vi "Helm Adjust Headings for PID.vi"(8 "error in (no error)":errorcluster, 11 "RDS Helm Actor in":refnum<class "RDS Helm Actor.lvclass">) -> (0 "error out":errorcluster, 1 "Current Position":dbl, 2 "Setpoint":dbl, 3 "RDS Helm Actor out":refnum<class "RDS Helm Actor.lvclass">)   [LabVIEW 2015, in "RDS Helm Actor.lvlib" / "RDS Helm Actor.lvclass"]
uses:
  RDS Helm Actor.lvclass
  RDS Helm Actor.lvclass/RDS Helm Actor.ctl
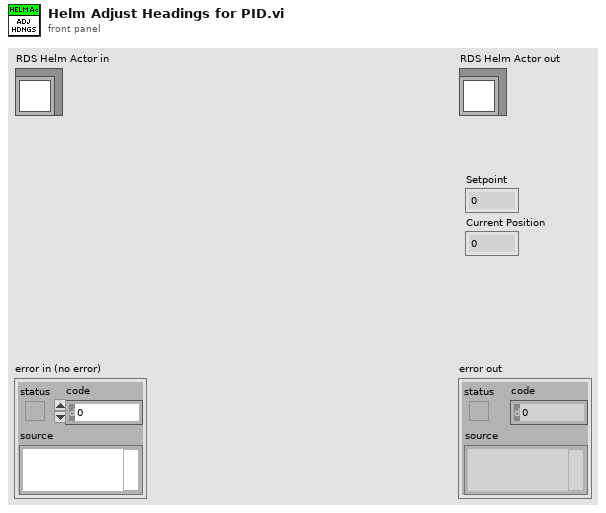
[diagram p1: front panel]
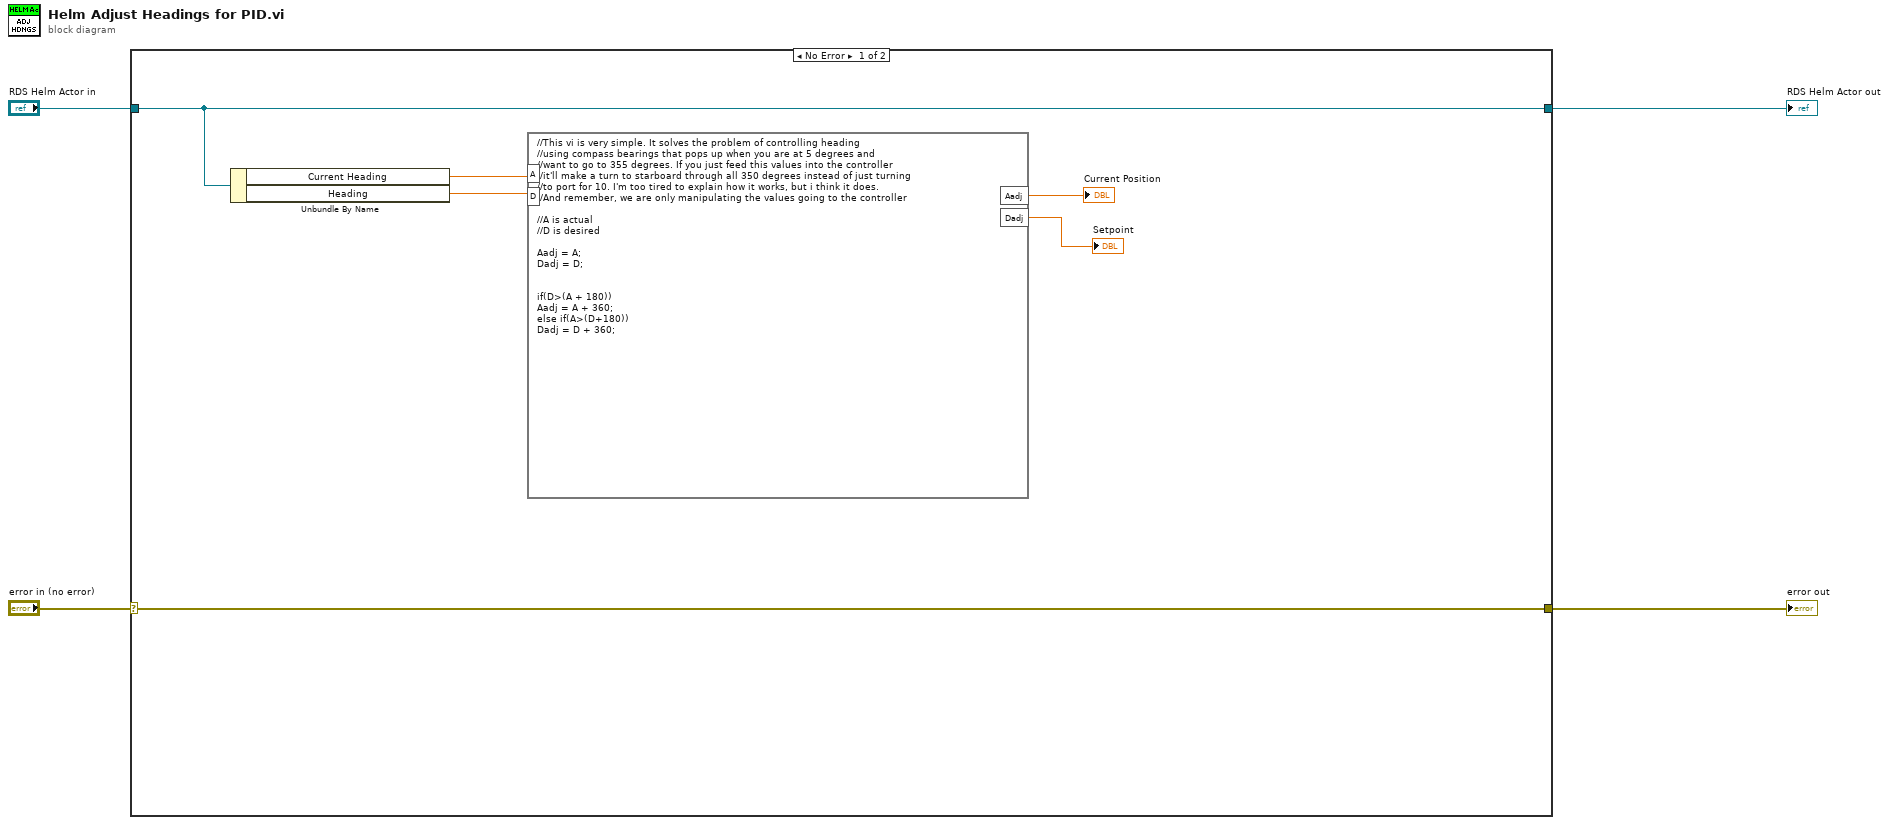
[diagram p0: block diagram]
diagram:
  n1 = case shown="No Error" "error in (no error)" {
    selector: "error in (no error)" -> [w10 w12]
    tunnel: [w10 w12] -> w3
    tunnel: [w9 w11] -> w1
    tunnel: "RDS Helm Actor in" -> [w9 w11]
    frame No Error {
      n2 = Unbundle By Name(w9) -> ("Current Heading"=w6:sgl, "Heading"=w5:sgl)
      n3 = formula code="//This vi is very simple. It solves the problem of controlling heading\n//using compass bearings that pops up when you are at 5 degrees and\n//want to go to 355 degrees. If you just feed this values into the controller\n//it'll make a turn to starboard through all 350 degrees instead of just turning\n//to port for 10. I'm too tired to explain how it works, but i think it does.\n//And remember, we are only manipulating the values going to the controller\n\n//A is actual\n//D is desired\n\nAadj = A;\nDadj = D;\n\n\nif(D>(A + 180))\nAadj = A + 360;\nelse if(A>(D+180))\nDadj = D + 360;"("A"=w6, "D"=w5) -> ("Aadj"=→"Current Position":dbl, "Dadj"=→"Setpoint":dbl)
    }
    frame Error {
    }
  }
  "error out" <- w3
  "RDS Helm Actor out" <- w1
